vi "UpdateCVT[Init].vi"(8 "error in (no error)":errorcluster, 11 "Photometrics Cam v2 in":refnum<class "Photometrics_CH-250_Cam.lvclass">) -> (0 "error out":errorcluster, 3 "Photometrics Cam v2 out":refnum<class "Photometrics_CH-250_Cam.lvclass">)   [LabVIEW 2013, in "Photometrics_CH-250_Cam.lvclass"]
doc: "Write the 'Init' data to the CVT"
uses:
  Photometrics_CH-250_Cam.lvclass
  shared/Cameras/GenericCameraClass/GenericCamera.lvclass
  Photometrics_CH-250_Cam.lvclass/Photometrics_CH-250_Cam.ctl
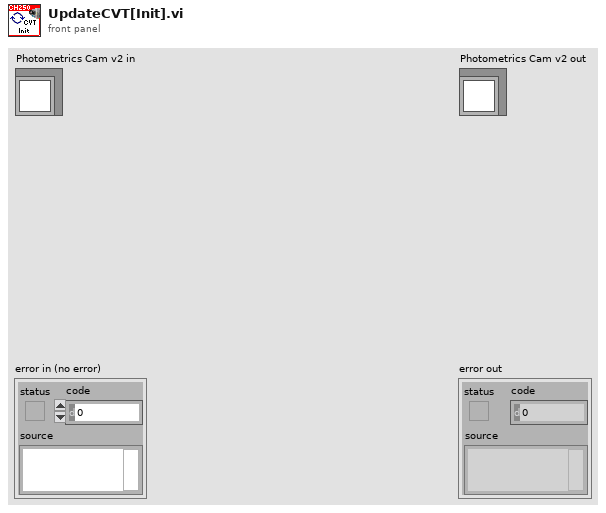
[diagram p1: front panel]
types:
  T1 = typedef "Photometrics_CH-250_Cam.lvclass/SettingsTypdef.ctl" = cluster{"trigger":T2, "gain":cluster{"Value":dbl, "Min":dbl, "Max":dbl, "StepSize":dbl, "Tolerance":dbl, "valueactual":dbl}, "Timeout":cluster{"Value":dbl, "Min":dbl, "Max":dbl, "StepSize":dbl, "Tolerance":dbl, "valueactual":dbl}, "localsavingpath":path, "save":T2, "camera name":string, "exposure":cluster{"Value":dbl, "Min":dbl, "Max":dbl, "StepSize":dbl, "Tolerance":dbl, "valueactual":dbl}, "TSetpoint":cluster{"Value":dbl, "Min":dbl, "Max":dbl, "StepSize":dbl, "Tolerance":dbl, "valueactual":dbl}, "TReading":cluster{"Value":dbl, "Min":dbl, "Max":dbl, "StepSize":dbl, "Tolerance":dbl, "valueactual":dbl}, "MaxGUIPixel":cluster{"Value":dbl, "Min":dbl, "Max":dbl, "StepSize":dbl, "Tolerance":dbl, "valueactual":dbl}, "GUIBinning":cluster{"Value":dbl, "Min":dbl, "Max":dbl, "StepSize":dbl, "Tolerance":dbl, "valueactual":dbl}, "ROI":T3, "pause":T2}
  T2 = typedef "OnOffTypeDef.ctl" = enum16{"off", "on"}
  T3 = typedef "ROI_TypDef.ctl" = cluster{"Width":cluster{"Value":dbl, "Min":dbl, "Max":dbl, "StepSize":dbl, "Tolerance":dbl, "valueactual":dbl}, "Height":cluster{"Value":dbl, "Min":dbl, "Max":dbl, "StepSize":dbl, "Tolerance":dbl, "valueactual":dbl}, "OffsetX":cluster{"Value":dbl, "Min":dbl, "Max":dbl, "StepSize":dbl, "Tolerance":dbl, "valueactual":dbl}, "OffsetY":cluster{"Value":dbl, "Min":dbl, "Max":dbl, "StepSize":dbl, "Tolerance":dbl, "valueactual":dbl}}
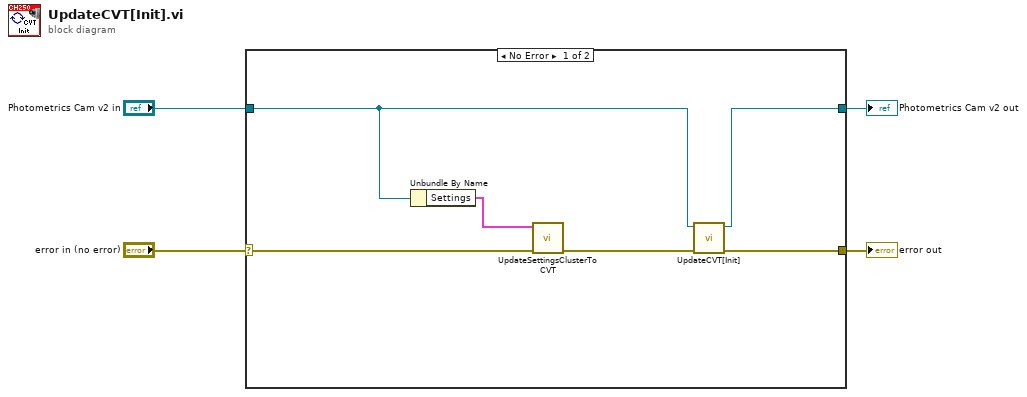
[diagram p0: block diagram]
diagram:
  n1 = case shown="No Error" "error in (no error)" {
    selector: "error in (no error)" -> [w9 w12]
    tunnel: [w5 w12] -> w3
    tunnel: [w6 w11] -> w1
    tunnel: "Photometrics Cam v2 in" -> [w7 w11]
    frame No Error {
      n2 = Unbundle By Name(w7) -> ("Settings"=w10:T1)
      n3 = call "UpdateSettingsClusterToCVT.vi"("error in (no error)"=w9, "variant"=w10) -> ("error out"=w8:errorcluster)  [unwired: 9 in]
      n4 = call-parent "UpdateCVT[Init].vi"("error in (no error)"=w8, "GenericCamera in"=w7) -> ("error out"=w5:errorcluster, "GenericCamera out"=w6:refnum<class "Photometrics_CH-250_Cam.lvclass">)  [unwired: 8 in]
    }
    frame Error {
    }
  }
  "error out" <- w3
  "Photometrics Cam v2 out" <- w1
